vi "Clear.vi"(8 "error in (no error)":errorcluster, 11 "Virtual Memory Unit in":refnum<class "Virtual Memory Unit.lvclass">) -> (0 "error out":errorcluster, 3 "Virtual Memory Unit out":refnum<class "Virtual Memory Unit.lvclass">)   [LabVIEW 2020, in "BCI-1553 API.lvlib" / "Virtual Memory.lvlib" / "Virtual Memory Unit.lvclass"]
doc: "Clears the entire contents of the Virtual Memory."
uses:
  Virtual Memory Unit.lvclass
  Virtual Memory Unit.lvclass/Virtual Memory Unit.ctl
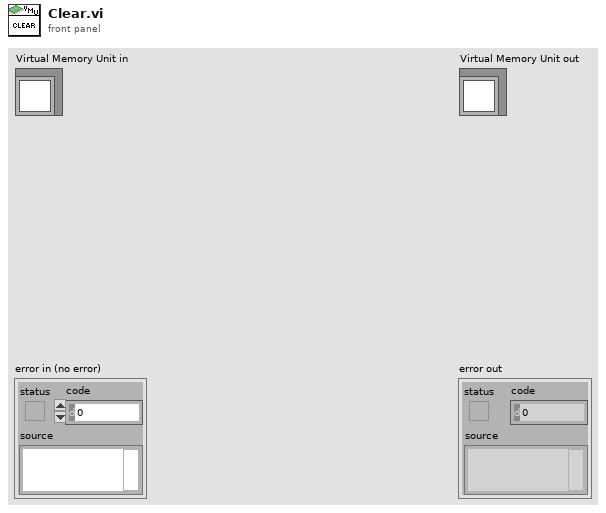
[diagram p1: front panel]
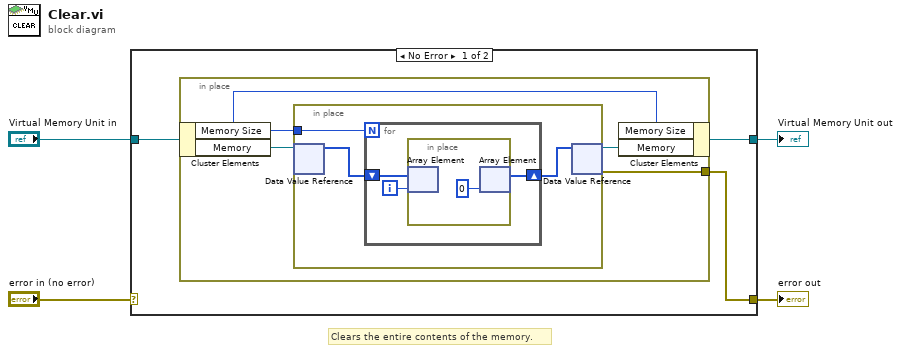
[diagram p0: block diagram]
diagram:
  # "Clears the entire contents of the memory."
  n1 = case shown="No Error" "error in (no error)" {
    selector: "error in (no error)" -> [_ w20]
    tunnel: [w5 w20] -> w3
    tunnel: [w6 w19] -> w1
    tunnel: "Virtual Memory Unit in" -> [w7 w19]
    frame No Error {
      n2 = in-place {
        in-place-border: [w8] -> w5
        n3 = in-place-cluster #1(w7) -> ("Memory Size"=w10:i32, "Memory"=w9:refnum<data-value>)
        n4 = in-place {
          in-place-border: w10 -> [w14]
          n5 = in-place-dvr #2(w9) -> (w13:u16[])  [unwired: 1 out]
          n6 = for {
            N: w14 -> [_]
            shift-right: [w15] -> w12
            shift-left: w13 -> [w17]
            i -> [w16]
            n7 = in-place {
              n8 = in-place-array #3(w17, w16) -> ()  [unwired: 1 out]
              n9 = in-place-array #3(u16 0) -> (w15:u16[])  [unwired: 1 out]
            }
          }
          n10 = in-place-dvr #2(w12) -> (w11:refnum<data-value>, w8:errorcluster)
        }
        n11 = in-place-cluster #1("Memory Size"=w10, "Memory"=w11) -> (w6:refnum<class "Virtual Memory Unit.lvclass">)
      }
    }
    frame Error {
    }
  }
  "error out" <- w3
  "Virtual Memory Unit out" <- w1
